vi "DisplaySettings 2 INI Section.vi"(8 "error in (no error)":errorcluster, 10 "Display settings":T2={"Min. Thresh."=0.0, "X"=0.0, "Y"=0.0, "ShowLineout"=FALSE, "ScaleParts"=10, "ShowLegende"=FALSE, "Target Cross"=FALSE, "Centroid Cross"=FALSE, "Target color"=16777226, "Centroid color"=16711680, "calibr. mm/px"=0.0}, 11 "refnum in":T1) -> (0 "error out":errorcluster, 3 "refnum out":T1)   [LabVIEW 2009, in "POLARIS IMAQ Display.xctl"]
uses:
  POLARIS IMAQ Display.xctl
  DisplaySettings.ctl
  <vilib>/Utility/config.llb/Config Data RefNum.ctl
  <vilib>/Utility/config.llb/Write Key (Double).vi
  <vilib>/Utility/config.llb/NI_LVConfig.lvlib
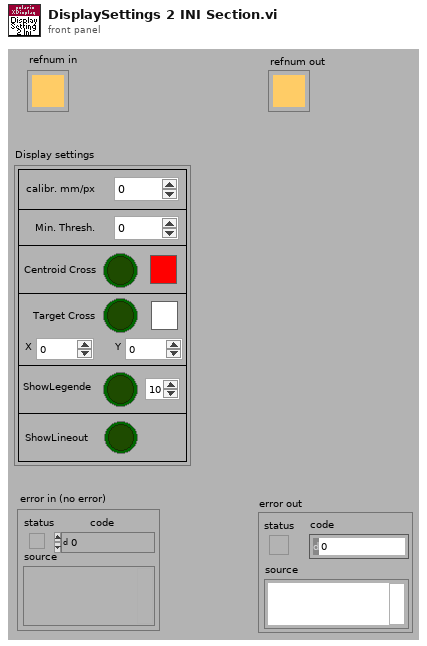
[diagram p1: front panel]
types:
  T1 = typedef "NI_LVConfig.lvlib/Config Data RefNum.ctl" = refnum<k1>
  T2 = typedef "POLARIS IMAQ Display.xctl/DisplaySettings.ctl" = cluster{"Min. Thresh.":sgl, "X":dbl, "Y":dbl, "ShowLineout":bool, "ScaleParts":i32, "ShowLegende":bool, "Target Cross":bool, "Centroid Cross":bool, "Target color":u32, "Centroid color":u32, "calibr. mm/px":sgl}
  T3 = enum16{"fractional", "engineering", "exponential"}
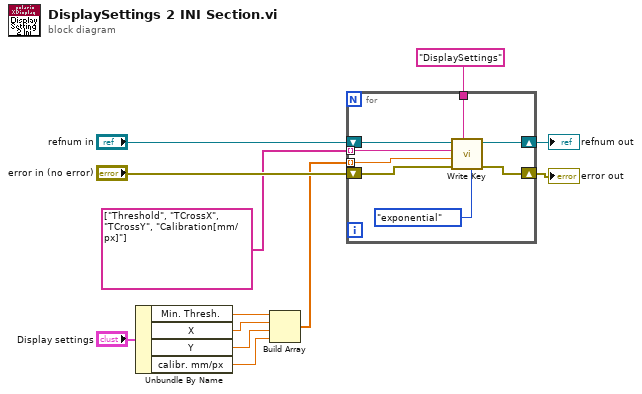
[diagram p0: block diagram]
diagram:
  n1 = Unbundle By Name("Display settings") -> ("Min. Thresh."=w8:sgl, "X"=w7:dbl, "Y"=w6:dbl, "calibr. mm/px"=w5:sgl)
  n2 = Build Array(w8, w7, w6, w5) -> (w2:dbl[])
  n3 = for {
    tunnel: "DisplaySettings" ("section") -> [w18]
    tunnel: w2 -> [w15] mode=indexing
    shift-right: [w16] -> w3
    shift-left: "error in (no error)" -> [w17]
    tunnel: string[] ["Threshold", "TCrossX", "TCrossY", "Calibration[mm/px]"] -> [w14] mode=indexing
    shift-right: [w19] -> w10
    shift-left: "refnum in" -> [w20]
    n4 = call-poly <vilib>:"Write Key.vi"("format (fractional)"=T3."exponential", "section"=w18, "error in (no error)"=w17, "value"=w15, "key"=w14, "refnum"=w20) -> ("error out"=w16:errorcluster, "refnum out"=w19:T1)  [unwired: 3 in, 1 out]
  }
  "refnum out" <- w10
  "error out" <- w3
